vi "Color Table To Reference.vi"(10 "Color Map":T1=enum."Red", 11 "Intensity Graph Reference":refnum<vi>) -> ()   [LabVIEW 2015]
uses:
  Type Defs/Color Map.ctl
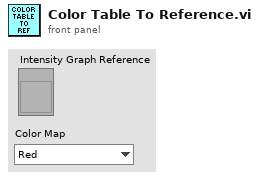
[diagram p1: front panel]
types:
  T1 = typedef "Color Map.ctl" = enum16{"Boring", "Fire", "Crazy", "Asylum", "Cubehelix", "Red", "Green", "Blue"}
  T2 = cluster{"ZScale.Minimum":dbl, "Z Scale.High Color":u32}
  T3 = cluster{"ZScale.Maximum":dbl, "Z Scale.High Color":u32}
  T4 = cluster{"ZScale.Minimum":dbl, "Z Scale.High Color":u32}[]
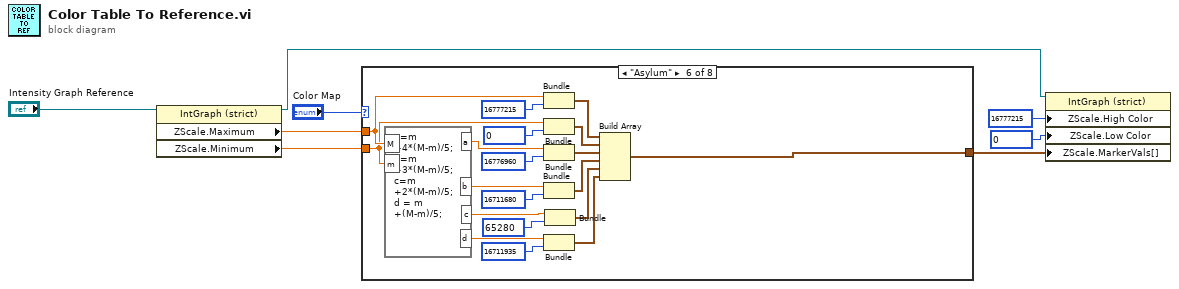
[diagram p0: block diagram]
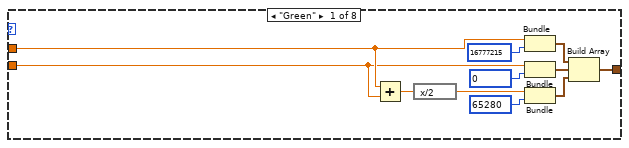
[diagram p2: hidden frame]
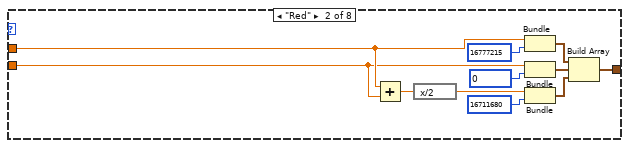
[diagram p3: hidden frame]
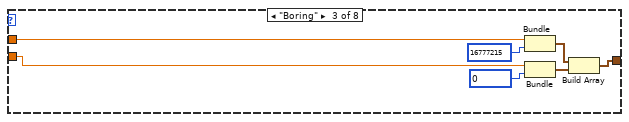
[diagram p4: hidden frame]
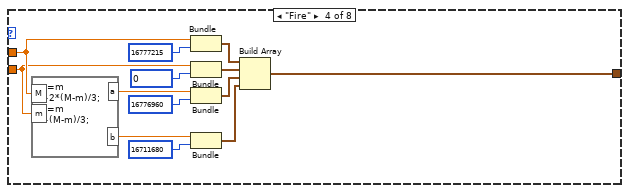
[diagram p5: hidden frame]
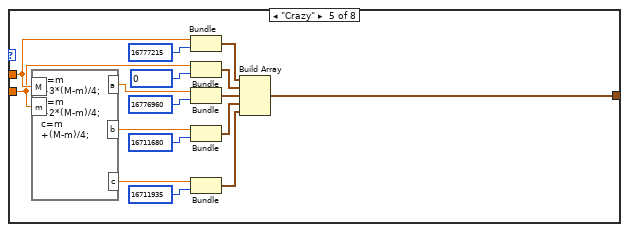
[diagram p6: hidden frame]
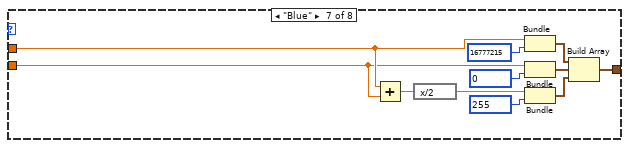
[diagram p7: hidden frame]
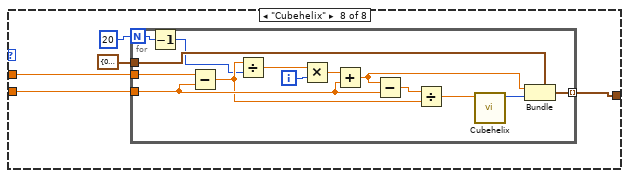
[diagram p8: hidden frame]
diagram:
  n1 = property class="IntGraph (strict)"(reference="Intensity Graph Reference") -> (reference out=w6:refnum<vi>, "ZScale.Maximum"=w5:dbl, "ZScale.Minimum"=w4:dbl)  [unwired: 1 in, 1 out]
  n2 = case shown="\"Asylum\"" "Color Map" {
    tunnel: w5 -> [w14 w25 w32 w41 w55 w75 w91 w98]
    tunnel: w4 -> [w13 w24 w31 w40 w54 w74 w90 w99]
    tunnel: [w19 w30 w37 w50 w66 w85 w96 w100] -> w3
    frame "Green" {
      n3 = Add(x=w14, y=w13) -> (x+y=w11:dbl)
      n4 = expression code="x/2"(w11) -> (w10:dbl)
      n5 = Bundle("ZScale.Maximum"=w14, "Z Scale.High Color"=u32 16777215) -> (w16:T3)  [unwired: 1 in]
      n6 = Bundle("ZScale.Minimum"=w13, "Z Scale.High Color"=u32 0) -> (w15:T2)  [unwired: 1 in]
      n7 = Bundle(w10, "Z Scale.High Color"=u32 65280) -> (w9:cluster{dbl, "Z Scale.High Color":u32})  [unwired: 1 in]
      n8 = Build Array(w16, w15, w9) -> (w19:T4)
    }
    frame "Red" {
      n9 = Add(x=w25, y=w24) -> (x+y=w22:dbl)
      n10 = expression code="x/2"(w22) -> (w21:dbl)
      n11 = Bundle("ZScale.Maximum"=w25, "Z Scale.High Color"=u32 16777215) -> (w27:T3)  [unwired: 1 in]
      n12 = Bundle("ZScale.Minimum"=w24, "Z Scale.High Color"=u32 0) -> (w26:T2)  [unwired: 1 in]
      n13 = Bundle(w21, "Z Scale.High Color"=u32 16711680) -> (w20:cluster{dbl, "Z Scale.High Color":u32})  [unwired: 1 in]
      n14 = Build Array(w27, w26, w20) -> (w30:T4)
    }
    frame "Boring" {
      n15 = Bundle("ZScale.Maximum"=w32, "Z Scale.High Color"=u32 16777215) -> (w34:T3)  [unwired: 1 in]
      n16 = Bundle("ZScale.Minimum"=w31, "Z Scale.High Color"=u32 0) -> (w33:T2)  [unwired: 1 in]
      n17 = Build Array(w34, w33) -> (w37:T4)
    }
    frame "Fire" {
      n18 = formula code="a=m\n+2*(M-m)/3;\nb=m\n+(M-m)/3;"("M"=w41, "m"=w40) -> ("a"=w39:dbl, "b"=w38:dbl)
      n19 = Bundle("ZScale.Maximum"=w41, "Z Scale.High Color"=u32 16777215) -> (w47:T3)  [unwired: 1 in]
      n20 = Bundle("ZScale.Minimum"=w40, "Z Scale.High Color"=u32 0) -> (w46:T2)  [unwired: 1 in]
      n21 = Bundle("a"=w39, "Z Scale.High Color"=u32 16776960) -> (w44:cluster{"a":dbl, "Z Scale.High Color":u32})  [unwired: 1 in]
      n22 = Bundle("b"=w38, "Z Scale.High Color"=u32 16711680) -> (w42:cluster{"b":dbl, "Z Scale.High Color":u32})  [unwired: 1 in]
      n23 = Build Array(w47, w46, w44, w42) -> (w50:cluster{"b":dbl, "Z Scale.High Color":u32}[])
    }
    frame "Crazy" {
      n24 = formula code="a=m\n+3*(M-m)/4;\nb=m\n+2*(M-m)/4;\nc=m\n+(M-m)/4;"("M"=w55, "m"=w54) -> ("a"=w53:dbl, "b"=w52:dbl, "c"=w51:dbl)
      n25 = Bundle("ZScale.Maximum"=w55, "Z Scale.High Color"=u32 16777215) -> (w63:T3)  [unwired: 1 in]
      n26 = Bundle("ZScale.Minimum"=w54, "Z Scale.High Color"=u32 0) -> (w62:T2)  [unwired: 1 in]
      n27 = Bundle("a"=w53, "Z Scale.High Color"=u32 16776960) -> (w60:cluster{"a":dbl, "Z Scale.High Color":u32})  [unwired: 1 in]
      n28 = Bundle("b"=w52, "Z Scale.High Color"=u32 16711680) -> (w58:cluster{"b":dbl, "Z Scale.High Color":u32})  [unwired: 1 in]
      n29 = Bundle("c"=w51, "Z Scale.High Color"=u32 16711935) -> (w56:cluster{"c":dbl, "Z Scale.High Color":u32})  [unwired: 1 in]
      n30 = Build Array(w63, w62, w60, w58, w56) -> (w66:cluster{"c":dbl, "Z Scale.High Color":u32}[])
    }
    frame "Asylum" {
      n31 = formula code="a=m\n+4*(M-m)/5;\nb=m\n+3*(M-m)/5;\nc=m\n+2*(M-m)/5;\nd = m\n+(M-m)/5;"("M"=w75, "m"=w74) -> ("a"=w73:dbl, "b"=w72:dbl, "d"=w71:dbl, "c"=w68:dbl)
      n32 = Bundle("ZScale.Maximum"=w75, "Z Scale.High Color"=u32 16777215) -> (w82:T3)  [unwired: 1 in]
      n33 = Bundle("ZScale.Minimum"=w74, "Z Scale.High Color"=u32 0) -> (w81:T2)  [unwired: 1 in]
      n34 = Bundle("a"=w73, "Z Scale.High Color"=u32 16776960) -> (w79:cluster{"a":dbl, "Z Scale.High Color":u32})  [unwired: 1 in]
      n35 = Bundle("b"=w72, "Z Scale.High Color"=u32 16711680) -> (w78:cluster{"b":dbl, "Z Scale.High Color":u32})  [unwired: 1 in]
      n36 = Bundle("d"=w71, "Z Scale.High Color"=u32 16711935) -> (w76:cluster{"d":dbl, "Z Scale.High Color":u32})  [unwired: 1 in]
      n37 = Bundle("c"=w68, "Z Scale.High Color"=u32 65280) -> (w67:cluster{"c":dbl, "Z Scale.High Color":u32})  [unwired: 1 in]
      n38 = Build Array(w82, w81, w79, w78, w67, w76) -> (w85:cluster{"d":dbl, "Z Scale.High Color":u32}[])
    }
    frame "Blue" {
      n39 = Add(x=w91, y=w90) -> (x+y=w88:dbl)
      n40 = expression code="x/2"(w88) -> (w87:dbl)
      n41 = Bundle("ZScale.Maximum"=w91, "Z Scale.High Color"=u32 16777215) -> (w93:T3)  [unwired: 1 in]
      n42 = Bundle("ZScale.Minimum"=w90, "Z Scale.High Color"=u32 0) -> (w92:T2)  [unwired: 1 in]
      n43 = Bundle(w87, "Z Scale.High Color"=u32 255) -> (w86:cluster{dbl, "Z Scale.High Color":u32})  [unwired: 1 in]
      n44 = Build Array(w93, w92, w86) -> (w96:T4)
    }
    frame "Cubehelix" {
      n45 = for {
        N: 20 -> [w112]
        tunnel: T2 {"ZScale.Minimum"=0.0, "Z Scale.High Color"=0} -> [w115]
        tunnel: [w114] -> w100 mode=indexing
        tunnel: w99 -> [w106]
        tunnel: w98 -> [w109]
        i -> [w110]
        n46 = Decrement(x=w112) -> (x-1=w102:i32)
        n47 = Subtract(x=w109, y=w106) -> (x-y=w104:dbl)
        n48 = Divide(x=w104, y=w102) -> (x/y=w111:dbl)
        n49 = Multiply(x=w111, y=w110) -> (x*y=w108:dbl)
        n50 = Add(x=w108, y=w106) -> (x+y=w107:dbl)
        n51 = Subtract(x=w107, y=w106) -> (x-y=w105:dbl)
        n52 = Divide(x=w105, y=w104) -> (x/y=w103:dbl)
        n53 = call "Cubehelix.vi"("Fraction (0 to 1)"=w103) -> ("RGB Hex Value"=w113:u32)  [unwired: 10 in]
        n54 = Bundle(cluster=w115, "ZScale.Minimum"=w107, "Z Scale.High Color"=w113) -> (w114:T2)
      }
    }
  }
  n55 = property class="IntGraph (strict)"(reference=w6, "ZScale.High Color"=u32 16777215 ("Z Scale.High Color"), "ZScale.Low Color"=u32 0 ("Z Scale.High Color"), "ZScale.MarkerVals[]"=w3) -> ()  [unwired: 1 in, 2 out]
